vi "FRAS Extraction imagettes.vi"(0 "Image 2":T1, 7 "Coordonnées_Images":sgl[][](array[numeric]), 11 "Longueur du coté":i32) -> (6 "Imagette1":i16[][](array[numeric]), 10 "Imagette2":i16[][](array[numeric]))   [LabVIEW 2020]
uses:
  <vilib>/vision/Image Controls.llb/IMAQ Image.ctl
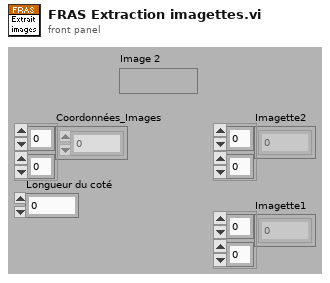
[diagram p1: front panel]
types:
  T1 = typedef "IMAQ Image.ctl" = refnum<image>
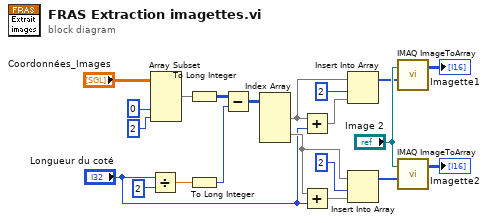
[diagram p0: block diagram]
diagram:
  n1 = Divide(x="Longueur du coté", y=2) -> (x/y=w4:dbl)
  n2 = Array Subset(array="Coordonnées_Images", index (col)=0 ("indice"), length (col)=2 ("longueur")) -> (w17:sgl[][])  [unwired: 2 in]
  n3 = To Long Integer(number=w17) -> (32bit integer=w6:i32[][])
  n4 = To Long Integer(number=w4) -> (32bit integer=w1:i32)
  n5 = Subtract(x=w6, y=w1) -> (x-y=w5:i32[][])
  n6 = Index Array(array=w5) -> (element #1=w8:i32[], element #2=w7:i32[])  [unwired: 4 in]
  n7 = Add(x=w8, y="Longueur du coté") -> (x+y=w13:i32[])
  n8 = Add(x=w7, y="Longueur du coté") -> (x+y=w10:i32[])
  n9 = Insert Into Array(array=w8, index=2 ("indice"), new element=w13) -> (w12:i32[])
  n10 = Insert Into Array(array=w7, index=2 ("indice"), new element=w10) -> (w9:i32[])
  n11 = call "IMAQ ImageToArray"("Optional Rectangle"=w12, "Image"="Image 2") -> ("Image Pixels (I16)"=→"Imagette1":i16[][])  [unwired: 1 in, 5 out]
  n12 = call "IMAQ ImageToArray"("Optional Rectangle"=w9, "Image"="Image 2") -> ("Image Pixels (I16)"=→"Imagette2":i16[][])  [unwired: 1 in, 5 out]
